vi "monitor get expected sync delta.vi"(11 "rate":u32(ring) items=["APDM_OUTPUT_SELECT_RATE_20", "APDM_OUTPUT_SELECT_RATE_32", "APDM_OUTPUT_SELECT_RATE_40", "APDM_OUTPUT_SELECT_RATE_64", "APDM_OUTPUT_SELECT_RATE_80", "APDM_OUTPUT_SELECT_RATE_128", "APDM_OUTPUT_SELECT_RATE_256", "APDM_OUTPUT_SELECT_RATE_512", "APDM_OUTPUT_SELECT_RATE_640", "APDM_OUTPUT_SELECT_RATE_1280"]) -> (3 "function return":u32)   [LabVIEW 2019, in "apdm.lvlib"]
doc: "APDM_EXPORT uint32_t apdm_monitor_get_expected_sync_delta(const apdm_monitor_output_select_rate_t rate);"
uses:
  apdm.lvlib
  Lee Lab/CP FES Walking 2018/Code/Working/LabVIEW/apdm.dll
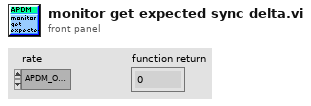
[diagram p1: front panel]
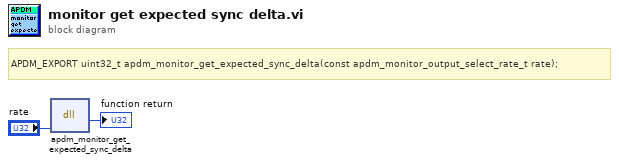
[diagram p0: block diagram]
diagram:
  # "APDM_EXPORT uint32_t apdm_monitor_get_expected_sync_delta(const apdm_monitor_output_select_rate_t rate);"
  n1 = dll-call lib="C:/Users/jfalesi/Dropbox/Lee Lab/CP FES Walking 2018/Code/Working/LabVIEW/apdm.*" fn="apdm_monitor_get_expected_sync_delta"("rate"="rate") -> (→"function return":u32)  [unwired: 4 in, 2 out]
